vi "create default alias.vi"(8 "error in":errorcluster, 11 "configuration in":refnum<class "Binary datalogger configuration.lvclass">) -> (0 "error out":errorcluster, 2 "default alias":string, 3 "configuration out":refnum<class "Binary datalogger configuration.lvclass">)   [LabVIEW 2013, in "Binary datalogger configuration.lvclass"]
uses:
  Binary datalogger configuration.lvclass
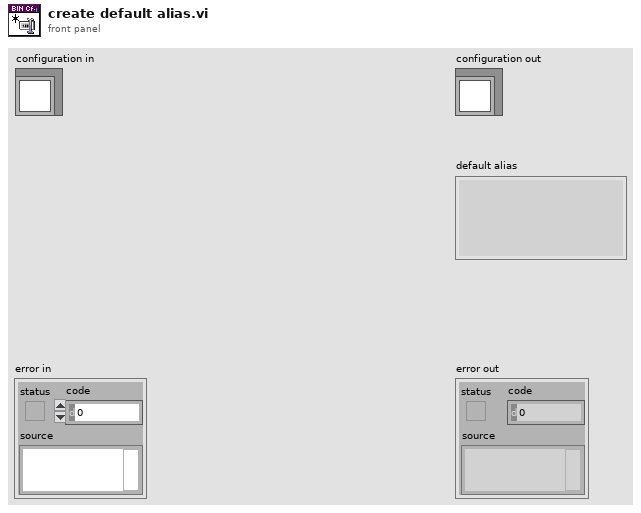
[diagram p1: front panel]
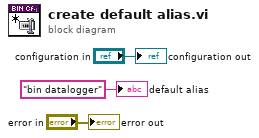
[diagram p0: block diagram]
diagram:
  "error out" <- "error in"
  "configuration out" <- "configuration in"
  "default alias" <- "bin datalogger" ("default alias")
